vi "Calcy_trial.vi"() -> ()   [LabVIEW 2025]
panel:
  out "String":string
  in  "0":bool
  in  "9":bool
  in  "8":bool
  in  "7":bool
  in  "6":bool
  in  "5":bool
  in  "4":bool
  in  "3":bool
  in  "2":bool
  in  "1":bool
  in  "Equ":bool
  in  "Div":bool
  in  "Mul":bool
  in  "Sub":bool
  in  "Add":bool
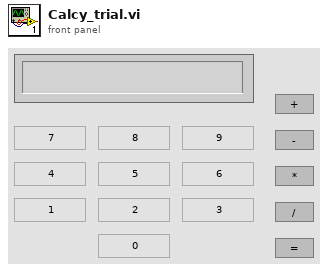
[diagram p1: front panel]
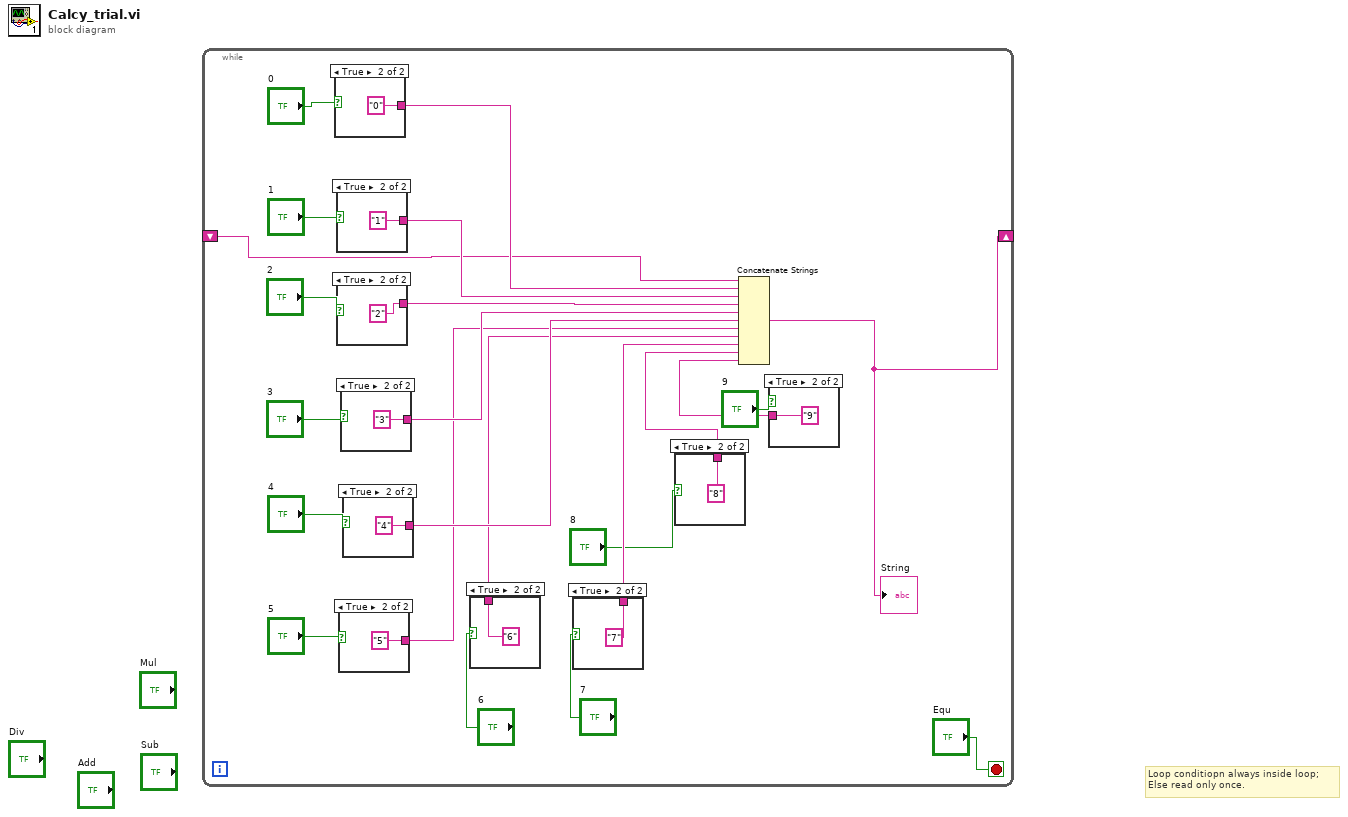
[diagram p0: block diagram]
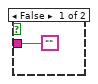
[diagram p2: hidden frame]
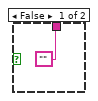
[diagram p3: hidden frame]
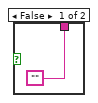
[diagram p4: hidden frame]
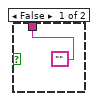
[diagram p5: hidden frame]
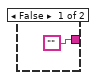
[diagram p6: hidden frame]
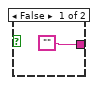
[diagram p7: hidden frame]
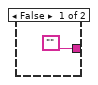
[diagram p8: hidden frame]
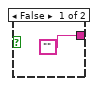
[diagram p9: hidden frame]
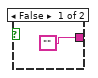
[diagram p10: hidden frame]
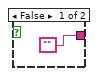
[diagram p11: hidden frame]
diagram:
  # "Loop conditiopn always inside loop;\nElse read only once."
  n1 = while {
    shift-right: [w2] -> _
    shift-left: _ -> [w1]
    stop <- "Equ" stop-if-true
    n2 = case shown="True" "0" {
      tunnel: ["" "0"] -> w5
      frame False {
      }
      frame True {
      }
    }
    n3 = case shown="True" "1" {
      tunnel: ["" "1"] -> w4
      frame False {
      }
      frame True {
      }
    }
    n4 = case shown="True" "2" {
      tunnel: ["" "2"] -> w20
      frame False {
      }
      frame True {
      }
    }
    n5 = case shown="True" "5" {
      tunnel: ["" "5"] -> w13
      frame False {
      }
      frame True {
      }
    }
    n6 = case shown="True" "3" {
      tunnel: ["" "3"] -> w18
      frame False {
      }
      frame True {
      }
    }
    n7 = case shown="True" "4" {
      tunnel: ["" "4"] -> w16
      frame False {
      }
      frame True {
      }
    }
    n8 = case shown="True" "6" {
      tunnel: ["" "6"] -> w12
      frame False {
      }
      frame True {
      }
    }
    n9 = case shown="True" "7" {
      tunnel: ["" "7"] -> w10
      frame False {
      }
      frame True {
      }
    }
    n10 = case shown="True" "8" {
      tunnel: ["" "8"] -> w8
      frame False {
      }
      frame True {
      }
    }
    n11 = case shown="True" "9" {
      tunnel: ["" "9"] -> w6
      frame False {
      }
      frame True {
      }
    }
    n12 = Concatenate Strings(w1, w5, w4, w20, w18, w16, w13, w12, w10, w8, w6) -> (w2:string)
    "String" <- w2
  }
